vi "Simulated Device FGV.vi"(11 "Request":string) -> (3 "Response":string)   [LabVIEW 2020]
uses:
  Controls/Device Code.ctl
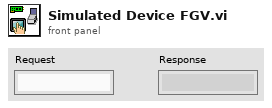
[diagram p1: front panel]
types:
  T1 = typedef "Device Code.ctl" = string
  T2 = cluster{"I/O Ports":cluster{"Port 0":bool[], "Port 1":bool[], "Port 2":bool[], "Port 3":bool[], "Port 4":bool[], "Port 5":bool[], "Port 6":bool[], "Port 7":bool[]}, "ADC Channels":cluster{"ADC Channel 1":u16, "ADC Channel 2":u16, "ADC Channel 3":u16, "ADC Channel 4":u16}}
  T3 = cluster{"Port 0":bool[], "Port 1":bool[], "Port 2":bool[], "Port 3":bool[], "Port 4":bool[], "Port 5":bool[], "Port 6":bool[], "Port 7":bool[]}
  T4 = cluster{"ADC Channel 1":u16, "ADC Channel 2":u16, "ADC Channel 3":u16, "ADC Channel 4":u16}
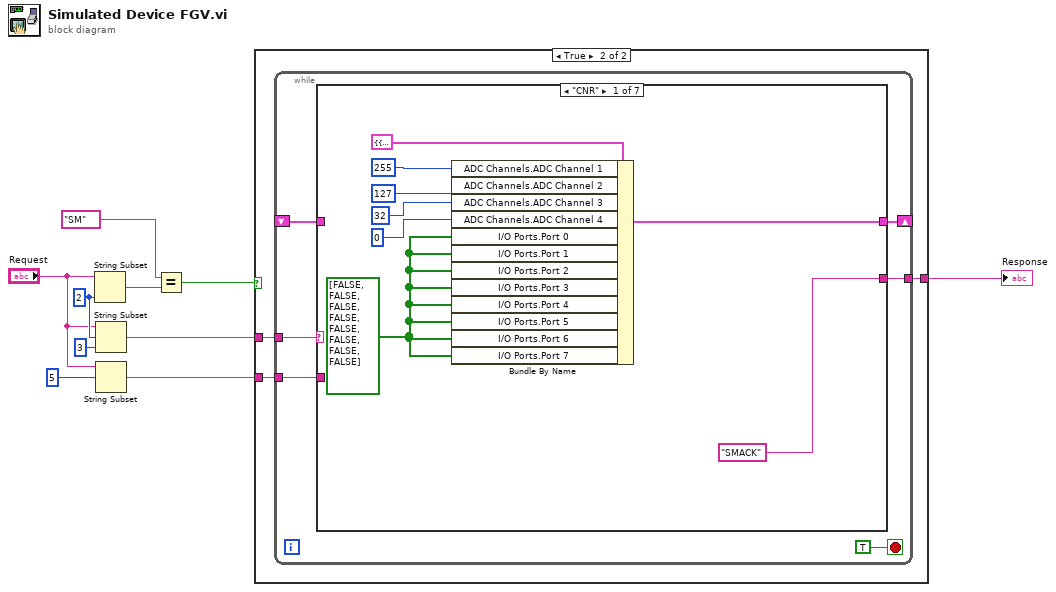
[diagram p0: block diagram]
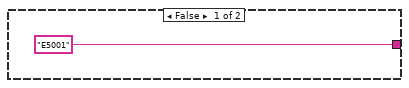
[diagram p2: hidden frame]
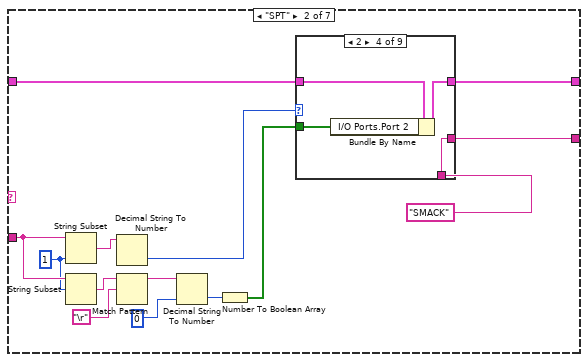
[diagram p3: hidden frame]
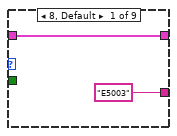
[diagram p4: hidden frame]
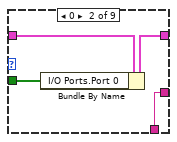
[diagram p5: hidden frame]
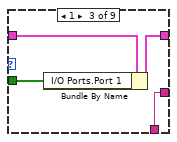
[diagram p6: hidden frame]
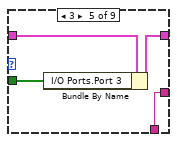
[diagram p7: hidden frame]
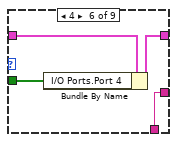
[diagram p8: hidden frame]
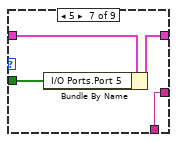
[diagram p9: hidden frame]
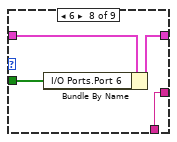
[diagram p10: hidden frame]
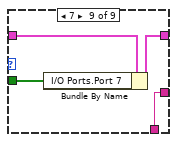
[diagram p11: hidden frame]
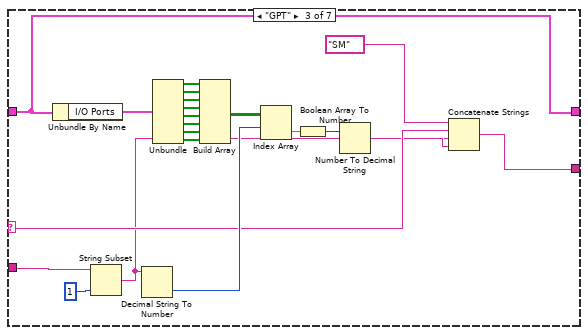
[diagram p12: hidden frame]
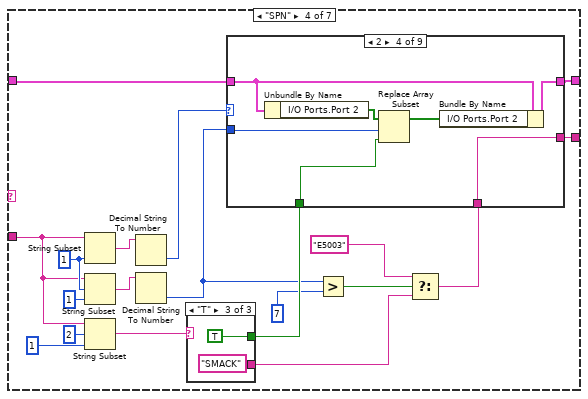
[diagram p13: hidden frame]
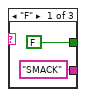
[diagram p14: hidden frame]
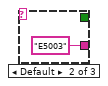
[diagram p15: hidden frame]
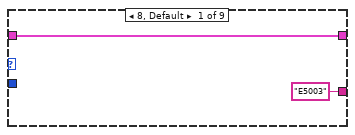
[diagram p16: hidden frame]
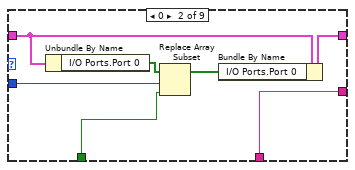
[diagram p17: hidden frame]
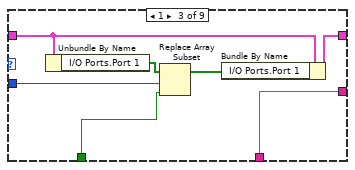
[diagram p18: hidden frame]
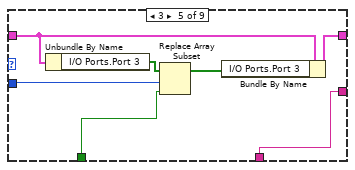
[diagram p19: hidden frame]
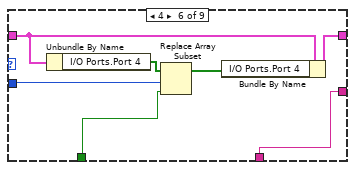
[diagram p20: hidden frame]
diagram:
  w6 = 2 ("length (rest)")
  n1 = String Subset(string="Request", length (rest)=w6) -> (substring=w7:string)  [unwired: 1 in]
  n2 = String Subset(string="Request", offset (0)=w6, length (rest)=3 ("length (rest)")) -> (substring=w4:string)
  n3 = String Subset(string="Request", offset (0)=5) -> (substring=w1:string)  [unwired: 1 in]
  n4 = Equal?(x=T1 "SM" ("Device Code"), y=w7) -> (x = y?=w9:bool)
  n5 = case shown="True" w9 {
    tunnel: ["E5001" w12] -> w8
    tunnel: w4 -> [_ w14]
    tunnel: w1 -> [_ w13]
    frame False {
    }
    frame True {
      n6 = while {
        tunnel: w14 -> [w16]
        tunnel: w13 -> [w15]
        shift-right: [w19] -> _
        shift-left: _ -> [w17]
        tunnel: [w18] -> w12
        stop <- TRUE stop-if-true
        n7 = case shown="\"CNR\"" w16 {
          selector: w16 -> [_ _ w82 _ w186 w207 _]
          tunnel: [w26 w33 w83 w112 w184 w205 w225] -> w19
          tunnel: ["SMACK" w30 w84 w102 w185 w209 "E5002"] -> w18
          tunnel: w17 -> [_ w34 w83 w113 w184 w205 w225]
          tunnel: w15 -> [_ w42 w81 w110 w183 w214 _]
          frame "CNR" {
            w21 = bool[] [FALSE, FALSE, FALSE, FALSE, FALSE, FALSE, FALSE, FALSE]
            n8 = Bundle By Name(cluster=T2 {"I/O Ports"={"Port 0"=[], "Port 1"=[], "Port 2"=[], "Port 3"=[], "Port 4"=[], "Port 5"=[], "Port 6"=[], "Port 7"=[]}, "ADC Channels"={"ADC Channel 1"=0, "ADC Channel 2"=0, "ADC Channel 3"=0, "ADC Channel 4"=0}} ("Simulated Device"), "ADC Channels.ADC Channel 1"=u16 255 ("ADC Channels.ADC Channel 4"), "ADC Channels.ADC Channel 2"=u16 127 ("ADC Channels.ADC Channel 4"), "ADC Channels.ADC Channel 3"=u16 32 ("ADC Channels.ADC Channel 4"), "ADC Channels.ADC Channel 4"=u16 0, "I/O Ports.Port 0"=w21, "I/O Ports.Port 1"=w21, "I/O Ports.Port 2"=w21, "I/O Ports.Port 3"=w21, "I/O Ports.Port 4"=w21, "I/O Ports.Port 5"=w21, "I/O Ports.Port 6"=w21, "I/O Ports.Port 7"=w21) -> (w26:T2)
          }
          frame "SPT" {
            w41 = 1 ("length (rest)")
            n9 = String Subset(string=w42, length (rest)=w41) -> (substring=w36:string)  [unwired: 1 in]
            n10 = String Subset(string=w42, offset (0)=w41) -> (substring=w40:string)  [unwired: 1 in]
            n11 = Decimal String To Number(string=w36) -> (number=w35:i32)  [unwired: 2 in, 1 out]
            n12 = Match Pattern(string=w40, regular expression="\r") -> (before substring=w38:string)  [unwired: 1 in, 3 out]
            n13 = Decimal String To Number(string=w38, default (0L)=u8 0 ("default (0 I32)")) -> (number=w32:u8)  [unwired: 1 in, 1 out]
            n14 = Number To Boolean Array(number=w32) -> (Boolean array=w31:bool[])
            n15 = case shown="2" w35 {
              tunnel: w34 -> [w44 w48 w52 w56 w60 w64 w68 w72 w76]
              tunnel: [w44 w47 w51 w55 w59 w63 w67 w71 w75] -> w33
              tunnel: w31 -> [_ w46 w50 w54 w58 w62 w66 w70 w74]
              tunnel: ["E5003" w45 w49 w53 w57 w61 w65 w69 w73] -> w30
              tunnel: "SMACK" -> [_ w45 w49 w53 w57 w61 w65 w69 w73]
              frame 8, Default {
              }
              frame 0 {
                n16 = Bundle By Name(cluster=w48, "I/O Ports.Port 0"=w46) -> (w47:T2)
              }
              frame 1 {
                n17 = Bundle By Name(cluster=w52, "I/O Ports.Port 1"=w50) -> (w51:T2)
              }
              frame 2 {
                n18 = Bundle By Name(cluster=w56, "I/O Ports.Port 2"=w54) -> (w55:T2)
              }
              frame 3 {
                n19 = Bundle By Name(cluster=w60, "I/O Ports.Port 3"=w58) -> (w59:T2)
              }
              frame 4 {
                n20 = Bundle By Name(cluster=w64, "I/O Ports.Port 4"=w62) -> (w63:T2)
              }
              frame 5 {
                n21 = Bundle By Name(cluster=w68, "I/O Ports.Port 5"=w66) -> (w67:T2)
              }
              frame 6 {
                n22 = Bundle By Name(cluster=w72, "I/O Ports.Port 6"=w70) -> (w71:T2)
              }
              frame 7 {
                n23 = Bundle By Name(cluster=w76, "I/O Ports.Port 7"=w74) -> (w75:T2)
              }
            }
          }
          frame "GPT" {
            n24 = Unbundle By Name(w83) -> ("I/O Ports"=w96:T3)
            n25 = String Subset(string=w81, length (rest)=1 ("length (rest)")) -> (substring=w77:string)  [unwired: 1 in]
            n26 = Decimal String To Number(string=w77) -> (number=w86:i32)  [unwired: 2 in, 1 out]
            n27 = Unbundle(w96) -> ("Port 0"=w95:bool[], "Port 1"=w94:bool[], "Port 2"=w93:bool[], "Port 3"=w92:bool[], "Port 4"=w91:bool[], "Port 5"=w90:bool[], "Port 6"=w89:bool[], "Port 7"=w88:bool[])
            n28 = Build Array(w95, w94, w93, w92, w91, w90, w89, w88) -> (w87:bool[][])
            n29 = Index Array(array=w87, index (row)=w86) -> (element=w80:bool[])  [unwired: 1 in]
            n30 = Boolean Array To Number(Boolean array=w80) -> (number=w79:u32)
            n31 = Number To Decimal String(number=w79) -> (decimal integer string=w78:string)  [unwired: 1 in]
            n32 = Concatenate Strings(T1 "SM" ("Device Code"), w82, w77, w78) -> (w84:string)
          }
          frame "SPN" {
            w116 = 1 ("length (rest)")
            n33 = String Subset(string=w110, length (rest)=w116) -> (substring=w115:string)  [unwired: 1 in]
            n34 = String Subset(string=w110, offset (0)=w116, length (rest)=1 ("length (rest)")) -> (substring=w107:string)
            n35 = String Subset(string=w110, offset (0)=2, length (rest)=1 ("length (rest)")) -> (substring=w106:string)
            n36 = Decimal String To Number(string=w115) -> (number=w114:i32)  [unwired: 2 in, 1 out]
            n37 = Decimal String To Number(string=w107) -> (number=w98:i32)  [unwired: 2 in, 1 out]
            n38 = case shown="\"T\"" w106 {
              tunnel: [FALSE _ TRUE] -> w105
              tunnel: ["SMACK" "E5003" "SMACK"] -> w104
              frame "F" {
              }
              frame Default {
              }
              frame "T" {
              }
            }
            n39 = Greater?(x=w98, y=7) -> (0:w100:bool)
            n40 = Select(t="E5003", s=w100, f=w104) -> (s? t:f=w103:string)
            n41 = case shown="2" w114 {
              tunnel: w113 -> [w122 w129 w135 w142 w146 w155 w162 w166 w174]
              tunnel: [w122 w130 w137 w144 w151 w158 w165 w172 w179] -> w112
              tunnel: w98 -> [_ w127 w134 w141 w147 w154 w161 w169 w175]
              tunnel: w105 -> [_ w126 w133 w140 w148 w153 w160 w168 w176]
              tunnel: w103 -> [_ w124 w131 w138 w150 w157 w164 w171 w178]
              tunnel: ["E5003" w124 w131 w138 w150 w157 w164 w171 w178] -> w102
              frame 8, Default {
              }
              frame 0 {
                n42 = Unbundle By Name(w129) -> ("I/O Ports.Port 0"=w128:bool[])
                n43 = Replace Array Subset(array=w128, new element=w126, index=w127) -> (w125:bool[])
                n44 = Bundle By Name(cluster=w129, "I/O Ports.Port 0"=w125) -> (w130:T2)
              }
              frame 1 {
                n45 = Unbundle By Name(w135) -> ("I/O Ports.Port 1"=w136:bool[])
                n46 = Replace Array Subset(array=w136, new element=w133, index=w134) -> (w132:bool[])
                n47 = Bundle By Name(cluster=w135, "I/O Ports.Port 1"=w132) -> (w137:T2)
              }
              frame 2 {
                n48 = Unbundle By Name(w142) -> ("I/O Ports.Port 2"=w143:bool[])
                n49 = Replace Array Subset(array=w143, new element=w140, index=w141) -> (w139:bool[])
                n50 = Bundle By Name(cluster=w142, "I/O Ports.Port 2"=w139) -> (w144:T2)
              }
              frame 3 {
                n51 = Unbundle By Name(w146) -> ("I/O Ports.Port 3"=w149:bool[])
                n52 = Replace Array Subset(array=w149, new element=w148, index=w147) -> (w145:bool[])
                n53 = Bundle By Name(cluster=w146, "I/O Ports.Port 3"=w145) -> (w151:T2)
              }
              frame 4 {
                n54 = Unbundle By Name(w155) -> ("I/O Ports.Port 4"=w156:bool[])
                n55 = Replace Array Subset(array=w156, new element=w153, index=w154) -> (w152:bool[])
                n56 = Bundle By Name(cluster=w155, "I/O Ports.Port 4"=w152) -> (w158:T2)
              }
              frame 5 {
                n57 = Unbundle By Name(w162) -> ("I/O Ports.Port 5"=w163:bool[])
                n58 = Replace Array Subset(array=w163, new element=w160, index=w161) -> (w159:bool[])
                n59 = Bundle By Name(cluster=w162, "I/O Ports.Port 5"=w159) -> (w165:T2)
              }
              frame 6 {
                n60 = Unbundle By Name(w166) -> ("I/O Ports.Port 6"=w170:bool[])
                n61 = Replace Array Subset(array=w170, new element=w168, index=w169) -> (w167:bool[])
                n62 = Bundle By Name(cluster=w166, "I/O Ports.Port 6"=w167) -> (w172:T2)
              }
              frame 7 {
                n63 = Unbundle By Name(w174) -> ("I/O Ports.Port 7"=w177:bool[])
                n64 = Replace Array Subset(array=w177, new element=w176, index=w175) -> (w173:bool[])
                n65 = Bundle By Name(cluster=w174, "I/O Ports.Port 7"=w173) -> (w179:T2)
              }
            }
          }
          frame "GPN" {
            w204 = 1 ("length (rest)")
            n66 = Unbundle By Name(w184) -> ("I/O Ports"=w202:T3)
            n67 = String Subset(string=w183, length (rest)=w204) -> (substring=w180:string)  [unwired: 1 in]
            n68 = Unbundle(w202) -> ("Port 0"=w201:bool[], "Port 1"=w200:bool[], "Port 2"=w199:bool[], "Port 3"=w198:bool[], "Port 4"=w197:bool[], "Port 5"=w196:bool[], "Port 6"=w195:bool[], "Port 7"=w194:bool[])
            n69 = String Subset(string=w183, offset (0)=w204, length (rest)=1 ("length (rest)")) -> (substring=w181:string)
            n70 = Decimal String To Number(string=w180) -> (number=w192:i32)  [unwired: 2 in, 1 out]
            n71 = Decimal String To Number(string=w181) -> (number=w191:i32)  [unwired: 2 in, 1 out]
            n72 = Build Array(w201, w200, w199, w198, w197, w196, w195, w194) -> (w193:bool[][])
            n73 = Index Array(array=w193, index (row)=w192, index (col)=w191) -> (element=w190:bool)
            n74 = Select(t="T", s=w190, f="F") -> (s? t:f=w182:string)
            n75 = Concatenate Strings(T1 "SM" ("Device Code"), w186, w180, w181, w182) -> (w185:string)
          }
          frame "ADC" {
            n76 = Unbundle By Name(w205) -> ("ADC Channels"=w213:T4)
            n77 = String Subset(string=w214, length (rest)=1 ("length (rest)")) -> (substring=w206:string)  [unwired: 1 in]
            n78 = Decimal String To Number(string=w206) -> (number=w208:i32)  [unwired: 2 in, 1 out]
            n79 = Cluster To Array(cluster=w213) -> (array=w210:u16[])
            n80 = Greater?(x=w208, y=3) -> (0:w211:bool)
            n81 = case shown="True" w211 {
              tunnel: w210 -> [w223 _]
              tunnel: [w218 "E5003"] -> w209
              tunnel: w208 -> [w222 _]
              tunnel: w207 -> [w219 _]
              tunnel: w206 -> [w216 _]
              frame False {
                n82 = Index Array(array=w223, index=w222) -> (element=w221:u16)
                n83 = Number To Decimal String(number=w221) -> (decimal integer string=w217:string)  [unwired: 1 in]
                n84 = Concatenate Strings(T1 "SM" ("Device Code"), w219, w216, w217) -> (w218:string)
              }
              frame True {
              }
            }
          }
          frame Default {
          }
        }
      }
    }
  }
  "Response" <- w8
